vi "close.vi"(8 "error in (no error)":errorcluster, 11 "MKS in":refnum<class "MKS.lvclass">) -> (0 "error out":errorcluster, 3 "MKS out":refnum<class "MKS.lvclass">)   [LabVIEW 2022 SP3, in "MKS.lvclass"]
uses:
  MKS.lvclass
  MKS.lvclass/MKS.ctl
  Pressure Monitor.lvclass
  <instrlib>/MKS 972B/MKS 972B.lvlib
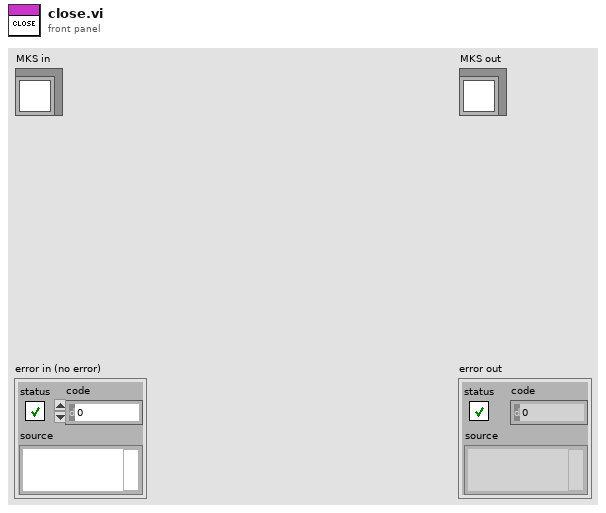
[diagram p1: front panel]
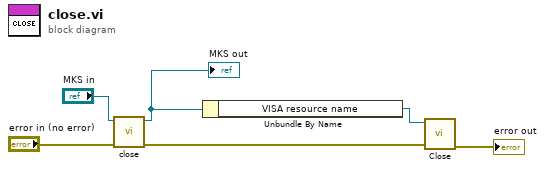
[diagram p0: block diagram]
diagram:
  n1 = call-parent <instrlib>:"close.vi"("error in (no error)"="error in (no error)", "Pressure Monitor in"="MKS in") -> ("error out"=w2:errorcluster, "Pressure Monitor out"=w4:refnum<class "MKS.lvclass">)  [unwired: 8 in]
  "MKS out" <- w4
  n2 = Unbundle By Name(w4) -> ("VISA resource name"=w3:refnum<visa-resource-name>)
  n3 = call <instrlib>:"Close.vi"("error in (no error)"=w2, "VISA resource name"=w3) -> ("error out"=→"error out":errorcluster)  [unwired: 9 in]
